vi "Wave Generation.vi"(0 "Pixel time (tick)":i32=80, 2 "Num of elements":u32=512000, 4 "Elements per line":i32=1000, 6 "Num of undershoot":i32=50, 7 "Resolution":i32=512, 8 "Pixel pulse_initial delay":i32=1, 9 "Pixel clock_pulse width(tick)":i32=40, 10 "Frame retrace time":u32=100 caption="Frame retrace time (ms)") -> (12 "Frame waveform output finish?":bool, 13 "Line clock":bool, 14 "Request address":u32, 16 "Galvo signal readed":u32, 17 "Data":u32, 19 "Pixel clock":bool)   [LabVIEW 2015]
uses:
  <vilib>/Platform/TimedLoop/XDataNode/timing_clust.ctl
  <vilib>/Platform/TimedLoop/XDataNode/nitl_modes.ctl
  <vilib>/Platform/TimedLoop/XDataNode/wakeup.ctl
  DRAM data index.ctl
  <vilib>/rvi/eio/common/nirviEmuTemplateMethod_errors.vi
  <vilib>/rvi/Emulation/niFpgaSctlEmulationGetInTimedLoop.vi
  <vilib>/rvi/Emulation/niFpgaEmulationReportErrorSimple.vi
  <vilib>/rvi/Emulation/niFpgaGetClockAttributes.vi
  <vilib>/rvi/Emulation/niFpgaCriticalErrorInLSC.vi
  <vilib>/rvi/Emulation/niFpgaProcessEmulError.vi
  <vilib>/eio/EIONode/EIONode.xnode
  <vilib>/Platform/TimedLoop/XDataNode/XDataNode.xnode
  <vilib>/Platform/TimedLoop/XDataNode/XDNodeRunTimeDep.lvlib
  Globals/Global_Sample per Frame.vi
panel:
  out "Numeric":i32
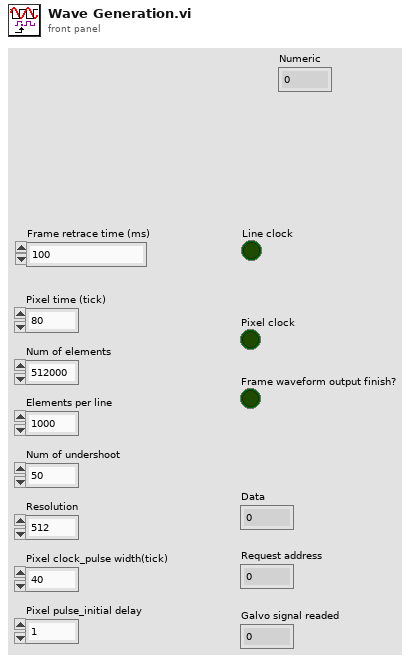
[diagram p1: front panel]
types:
  T1 = typedef "XDNodeRunTimeDep.lvlib/timing_clust.ctl" = cluster{"Expected End [f-1]":u64, "Actual End [f-1]":u64, "Finished Late? [f-1]":bool, "Expected End [i-1]":u64, "Actual End [i-1]":u64, "Finished Late? [i-1]":bool, "Expected Start [i]":u64, "Actual Start [i]":u64, "Expected Start [f]":u64, "Actual Start [f]":u64, "Source Name":string, "Structure Name":string, "Period":i64, "Deadline":i64, "Offset":i64, "Start":i64, "Priority":i32, "Timeout":i32, "Mode":T2, "Wakeup Reason":T3, "Error":errorcluster, "Source Type":string, "Secondary Source Type":string, "Global End Time":u64, "Global Start Time":u64, "Frame Duration":u64, "Iteration Duration":u64, "Assigned CPU":i32, "I/O Scan Engine Mode":u32}
  T2 = typedef "XDNodeRunTimeDep.lvlib/nitl_modes.ctl" = enum32{"No Change", "Process missed periods, maintain original phase", "Discard missed periods, maintain original phase", "Process missed periods, ignore original phase", "Discard missed periods, ignore original phase"}
  T3 = typedef "XDNodeRunTimeDep.lvlib/wakeup.ctl" = enum32{"Normal", "Aborted", "Asynchronous wakeup", "Timing source error", "Timed loop error", "Timeout"}
  T4 = typedef "DRAM data index.ctl" = enum16{"Numeric 1", "Numeric 2", "Numeric 3", "Numeric 4", "Numeric 5", "Numeric 6", "Numeric 7", "Numeric 8", "Numeric 9", "Numeric 10", "Numeric 11", "Numeric 12", "Numeric 13", "Numeric 14", "Numeric 15", "Numeric 16"}
  T5 = cluster{"Numeric 1":u32, "Numeric 2":u32, "Numeric 3":u32, "Numeric 4":u32, "Numeric 5":u32, "Numeric 6":u32, "Numeric 7":u32, "Numeric 8":u32, "Numeric 9":u32, "Numeric 10":u32, "Numeric 11":u32, "Numeric 12":u32, "Numeric 13":u32, "Numeric 14":u32, "Numeric 15":u32, "Numeric 16":u32}
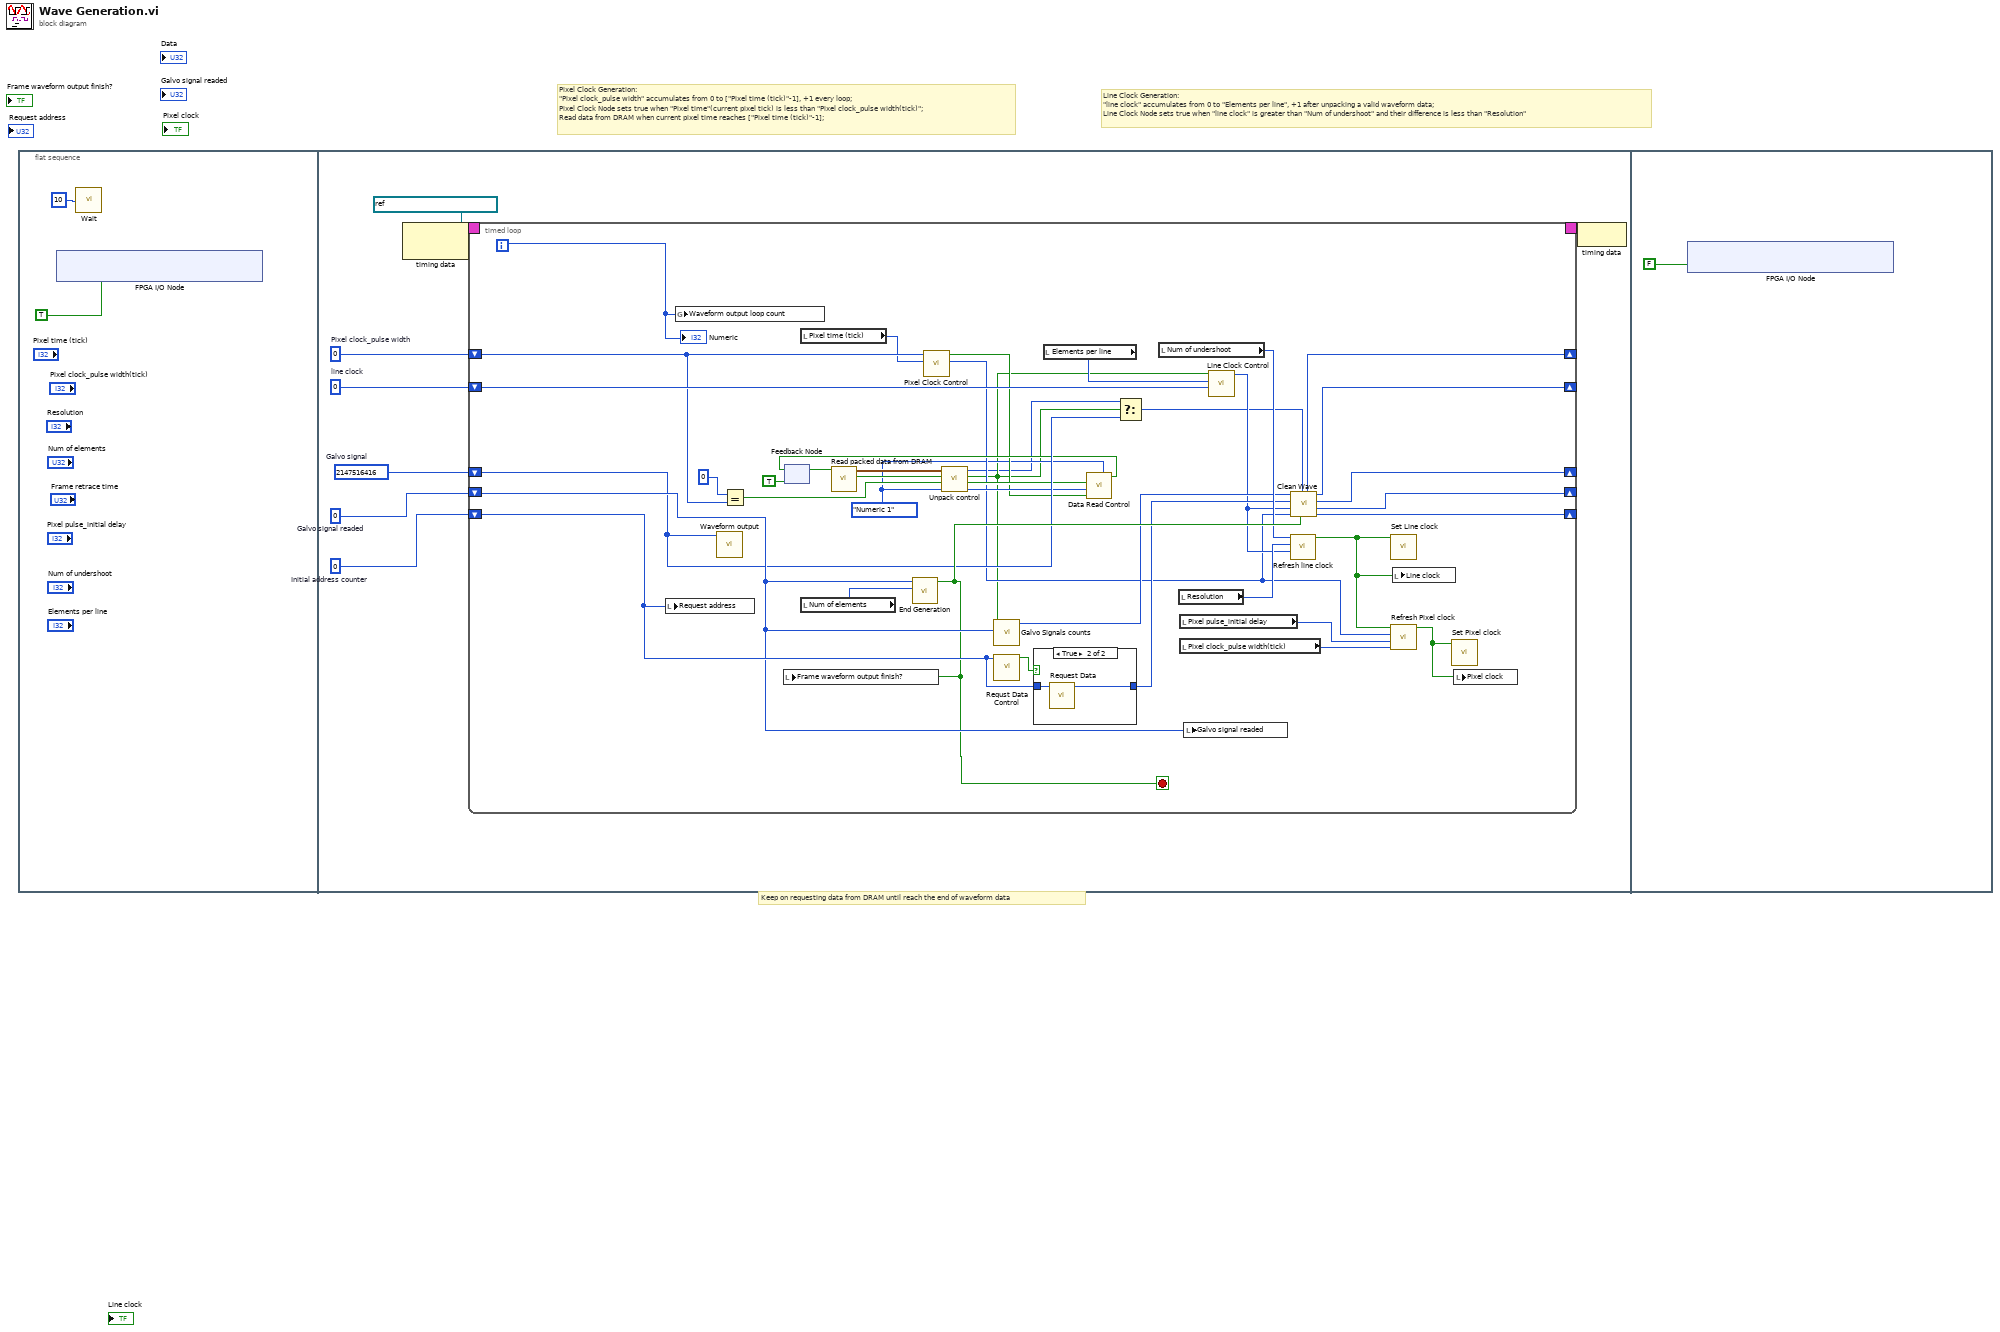
[diagram p0: block diagram]
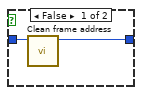
[diagram p2: hidden frame]
diagram:
  # "Keep on requesting data from DRAM until reach the end of waveform data"
  # "Line Clock Generation:\n\"line clock\" accumulates from 0 to \"Elements per line\", +1 after unpacking a valid waveform data;\nLine Clock Node sets true when \"line clock\" is greater than \"Num of undershoot\" and their difference is less than \"Resolution\""
  # "Pixel Clock Generation: \n\"Pixel clock_pulse width\" accumulates from 0 to [\"Pixel time (tick)\"-1], +1 every loop;\nPixel Clock Node sets true when \"Pixel time\"(current pixel tick) is less than \"Pixel clock_pulse width(tick)\";\nRead data from DRAM when current pixel time reaches [\"Pixel time (tick)\"-1];"
  n1 = flat-sequence {
    frame #0 {
      n2 = xnode "FPGA I/O Node"("IO Module\\Shutter(DDCA_PFI1_WRITE)"=TRUE ("IO Module\\Shutter(DDCA_PFI1_WRITE)")) -> ()  [unwired: 1 in, 1 out]
      n3 = call "Wait"("Count(uSec)"=u32 10) -> ()  [unwired: 1 out]
    }
    frame #1 {
      w7 = u32 0  # Initial address counter
      w4 = 0  # Pixel clock_pulse width
      w5 = 0  # line clock
      w6 = u32 0  # Galvo signal readed
      w3 = u32 2147516416  # Galvo signal
      n4 = node-c288(refnum<k21> "40 MHz Onboard Clock" ("Source Name")) -> (w10:T1)
      n5 = timed-loop {
        timing: w10 -> [_]
        timing-out: [_] -> w9
        shift-right: [w43] -> _
        shift-left: w7 -> [w49]
        shift-right: [w46] -> _
        shift-left: w3 -> [w41]
        shift-right: [w45] -> _
        shift-left: w6 -> [w47]
        shift-right: [w44] -> _
        shift-left: w5 -> [w50]
        shift-right: [w40] -> _
        shift-left: w4 -> [w48]
        i -> [w39]
        stop <- w42 stop-if-true
        w14 = DRAM_data_index."Numeric 1" ("DRAM pack index out")
        n6 = local write "Request address"(w49) -> ()
        n7 = global write "Global_Sample per Frame.vi" "Waveform output loop count"(w39) -> ()
        n8 = call "Waveform output.vi"("Galvo signal"=w41) -> ()  [unwired: 11 in]
        n9 = Equal?(x=0, y=w48) -> (x = y?=w31:bool)
        n10 = feedback #1(TRUE) -> (w33:bool)
        n11 = local read "Pixel time (tick)"() -> (w30:i32)
        n12 = local read "Num of elements"() -> (w26:u32)
        n13 = call "Read packed data from DRAM.vi"("Output ready"=w33) -> ("Output Valid§"=w37:bool, "Data"=w36:T5)  [unwired: 9 in]
        n14 = call "End Generation.vi"("Num of elements"=w26, "Galvo signal readed"=w47) -> ("End Generation"=w42:bool)  [unwired: 9 in]
        n15 = local write "Frame waveform output finish?"(w42) -> ()
        n16 = call "Pixel Clock Control.vi"("Pixel time (tick)"=w30, "Pixel clock_pulse width"=w48) -> ("Pixel time"=w16:i32, "Pixel time up"=w15:bool)  [unwired: 8 in]
        n17 = call "Unpack control.vi"("DRAM pack index init"=w14, "enable unpack"=w31, "input valid"=w37, "Data"=w36) -> ("output valid?"=w29:bool, "output valid? 2"=w13:bool, "Unpacked data"=w12:u32, "DRAM pack index out out"=w27:T4)  [unwired: 4 in]
        n18 = call "Galvo Signals counts.vi"("Galvo signal readed in"=w47, "output valid? in"=w13) -> ("Galvo signal readed out"=w19:u32)  [unwired: 9 in]
        n19 = call "Requst Data Control.vi"("Initial address counter"=w49) -> ("Enable request"=w34:bool)  [unwired: 10 in]
        n20 = case shown="True" w34 {
          tunnel: w49 -> [w51 w54]
          tunnel: [w52 w53] -> w18
          frame False {
            n21 = call "Clean frame address.vi"("Initial address counter in"=w51) -> ("Initial address counter out"=w52:u32)  [unwired: 10 in]
          }
          frame True {
            n22 = call "Request Data.vi"("Address counter"=w54) -> ("Address counter output"=w53:u32)  [unwired: 10 in]
          }
        }
        n23 = local read "Elements per line"() -> (w38:i32)
        n24 = call "Data Read Control.vi"("DRAM pack index out"=w14, "Pixel time up"=w15, "DRAM pack index out out"=w27, "input valid?"=w29) -> ("output valid"=w28:bool)  [unwired: 7 in]
        n25 = feedback-in #1(w28) -> ()
        n26 = Select(t=w12, s=w13, f=w41) -> (s? t:f=w11:u32)
        n27 = local read "Num of undershoot"() -> (w24:i32)
        n28 = local read "Resolution"() -> (w25:i32)
        n29 = local read "Pixel pulse_initial delay"() -> (w22:i32)
        n30 = local read "Pixel clock_pulse width(tick)"() -> (w21:i32)
        n31 = local write "Galvo signal readed"(w47) -> ()
        n32 = call "Line Clock Control.vi"("line clock in"=w50, "Elements per line"=w38, "output valid? in"=w13) -> ("line clock out"=w17:i32)  [unwired: 8 in]
        n33 = call "Refresh line clock.vi"("line clock output"=w17, "Resolution"=w25, "Num of undershoot"=w24) -> ("Refresh?"=w23:bool)  [unwired: 8 in]
        n34 = call "Clean Wave.vi"("line clock out"=w17, "Galvo signal in"=w11, "pixel clock_pulse width in"=w16, "Clean wave"=w42, "Address counter output"=w18, "Galvo signal readed out"=w19) -> ("Address counter"=w43:u32, "Galvo signal readed out"=w45:u32, "Galvo signal in"=w46:u32, "line clock"=w44:i32, "pixel clock_pulse width out"=w40:i32)  [unwired: 1 in]
        n35 = call "Set Line clock.vi"("Refresh"=w23) -> ()  [unwired: 11 in]
        n36 = call "Refresh Pixel clock.vi"("Pixel clock_pulse width(tick)"=w21, "Pixel pulse_initial delay"=w22, "Pixel clock_pulse width"=w16, "Refresh input"=w23) -> ("Refresh output"=w20:bool)  [unwired: 7 in]
        n37 = local write "Line clock"(w23) -> ()
        n38 = call "Set Pixel clock.vi"("Refresh"=w20) -> ()  [unwired: 11 in]
        n39 = local write "Pixel clock"(w20) -> ()
        "Numeric" <- w39
      }
      n40 = node-c288(w9) -> ()
    }
    frame #2 {
      n41 = xnode "FPGA I/O Node"("IO Module\\Shutter(DDCA_PFI1_WRITE)"=FALSE ("IO Module\\Shutter(DDCA_PFI1_WRITE)")) -> ()  [unwired: 1 in, 1 out]
    }
  }
